vi "Deque Traces.vi"(6 "Timeout [s]":dbl=10.0, 8 "error in (no error)":errorcluster, 10 "Averaging":T2 {"Traces" min=1 max=200 step=1}, 11 "Acquired Traces Queue":refnum<queue>) -> (0 "error out":errorcluster, 2 "Traces":waveform(sgl)[][](array[waveform]), 3 "Latest Acquisition Result":T1 {"Update rate [1/s]" format="%_3p"})   [LabVIEW 2019]
uses:
  Averaging.ctl
  Controls/Acquisition Result.ctl
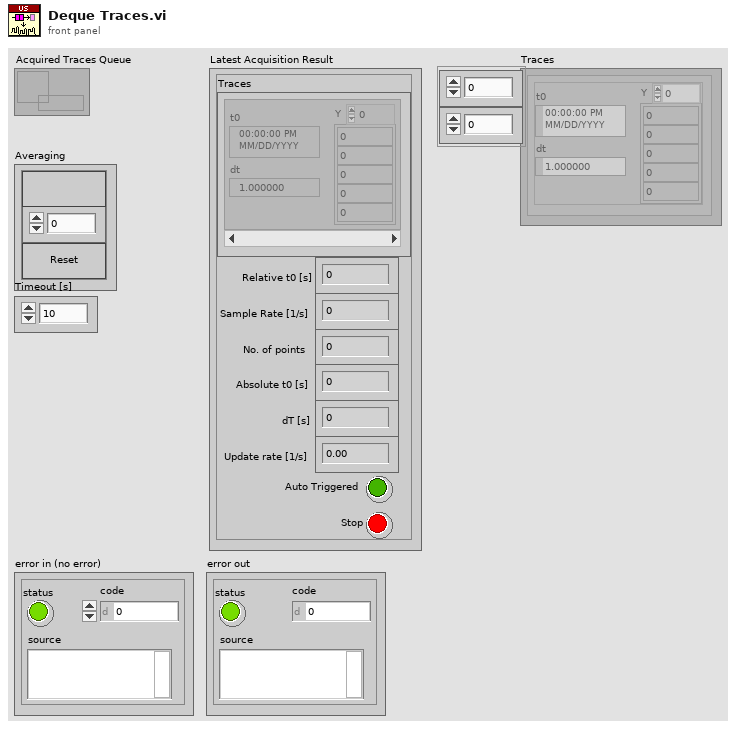
[diagram p1: front panel]
types:
  T1 = typedef "Acquisition Result.ctl" = cluster{"Traces":waveform(sgl)[], "Relative t0 [s]":dbl, "Sample Rate [1/s]":dbl, "No. of points":i32, "Absolute t0 [s]":dbl, "dT [s]":dbl, "Update rate [1/s]":dbl, "Auto Triggered":bool, "Stop":bool}
  T2 = typedef "Averaging.ctl" = cluster{"On":bool, "Traces":i32, "Reset":bool}
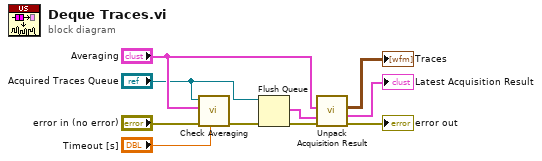
[diagram p0: block diagram]
diagram:
  n1 = call "Check Averaging.vi"("Timeout [s]"="Timeout [s]", "Error In"="error in (no error)", "Averaging"="Averaging", "Result Queue"="Acquired Traces Queue") -> ("Error Out"=w8:errorcluster)  [unwired: 6 in, 1 out]
  n2 = Flush Queue(queue="Acquired Traces Queue", error in (no error)=w8) -> (remaining elements=w5:T1[], error out=w3:errorcluster)  [unwired: 1 out]
  n3 = call "Unpack Acquisition Result.vi"("Error In"=w3, "Acquisition Results"=w5, "Averaging"="Averaging") -> ("Error Out"=→"error out":errorcluster, "Last Acquisition Result"=→"Latest Acquisition Result":T1, "Traces"=→"Traces":waveform(dbl)[][])  [unwired: 6 in]
